vi "Fetch Multi Eval Meas List TPower Results.vi"(8 "error in (no error)":errorcluster, 9 "Result Type (Current)":i32(ring) items=["Current"=0, "Average"=1, "Standard Deviation"=3, "Maximum"=4, "Minimum"=5], 10 "Instance (1)":T1=1, 11 "VISA resource name":refnum<visa-resource-name>) -> (0 "error out":errorcluster, 1 "TPower Results":dbl[](array[numeric]) format="%^.3e", 2 "Reliability":i32, 3 "VISA resource name out":refnum<visa-resource-name>)   [LabVIEW 2015, in "Rohde&Schwarz CMXP NR FR2 Measurement.lvlib"]
doc: "Returns user equipment power values for all measured list mode segments.\n\nAttributes:\nRSCMXPNRFR2M_ATTR_FETCH_MULTI_EVAL_MEASUREMENT_LIST_TPOWER_AVERAGE_RESULTS\nRSCMXPNRFR2M_ATTR_FETCH_MULTI_EVAL_MEASUREMENT_LIST_TPOWER_CURRENT_RESULTS\nRSCMXPNRFR2M_ATTR_FETCH_MULTI_EVAL_MEASUREMENT_LIST_TPOWER_MAXIMUM_RESULTS\nRSCMXPNRFR2M_ATTR_FETCH_MULTI_EVAL_MEASUREMENT_LIST_TPOWER_MINIMUM_RESULTS\nRSCMXPNRFR2M_ATTR_FETCH_MULTI_EVAL_MEASUREMENT_LIST_TPOWER_STANDARD_DEVIATION_RESULTS\n\nRemote-control commands:\nFETCh:NRMMw:MEAS<i>:MEValuation:LIST:MODulation:TPOWer:AVERage?\nFETCh:NRMMw:MEAS<i>:MEValuation:LIST:MODulation:TPOWer:CURRent?\nFETCh:NRMMw:MEAS<i>:MEValuation:LIST:MODulation:TPOWer:MAXimum?\nFETCh:NRMMw:MEAS<i>:MEValuation:LIST:MODulation:TPOWer:MINimum?\nFETCh:NRMMw:MEAS<i>:MEValuation:LIST:MODulation:TPOWer:SDEViation?"
uses:
  <instrlib>/Rohde&Schwarz CMXP NR FR2 Measurement/Rohde&Schwarz CMXP NR FR2 Measurement.lvlib
  <instrlib>/Rohde&Schwarz CMXP NR FR2 Measurement/Private/_Instance.ctl
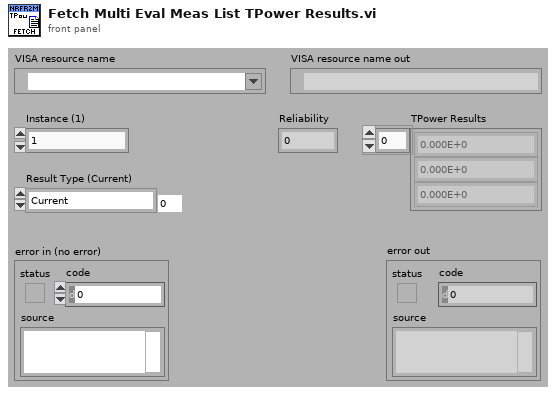
[diagram p1: front panel]
types:
  T1 = typedef "Rohde&Schwarz CMXP NR FR2 Measurement.lvlib/_Instance.ctl" = i32
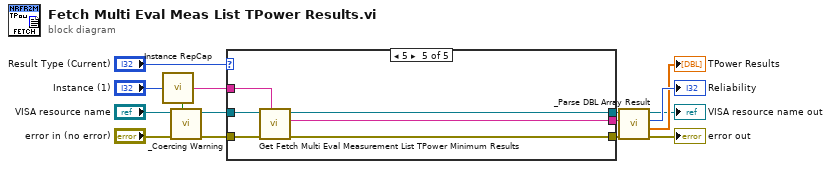
[diagram p0: block diagram]
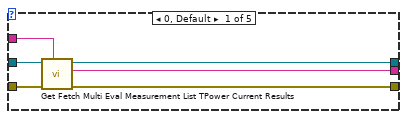
[diagram p2: hidden frame]
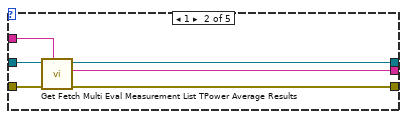
[diagram p3: hidden frame]
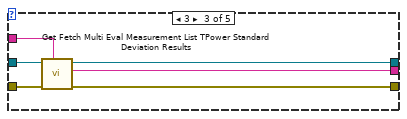
[diagram p4: hidden frame]
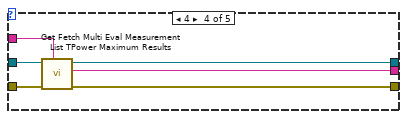
[diagram p5: hidden frame]
diagram:
  n1 = call <instrlib>:"Instance RepCap.vi"("Instance In"="Instance (1)") -> ("In Range?"=w13:bool, "RepCap Identifier Out"=w10:string)  [unwired: 1 in]
  n2 = call <instrlib>:"_Coercing Warning.vi"("In Range?"=w13, "error in (no error)"="error in (no error)", "VISA resource name"="VISA resource name") -> ("error out"=w12:errorcluster, "VISA resource name out"=w11:refnum<visa-resource-name>)  [unwired: 7 in]
  n3 = case shown="5" "Result Type (Current)" {
    tunnel: w12 -> [w21 w27 w33 w39 w45]
    tunnel: w11 -> [w20 w26 w32 w38 w44]
    tunnel: w10 -> [w19 w25 w31 w37 w43]
    tunnel: [w18 w24 w30 w36 w42] -> w8
    tunnel: [w17 w23 w29 w35 w41] -> w7
    tunnel: [w16 w22 w28 w34 w40] -> w6
    frame 0, Default {
      n4 = call "Get Fetch Multi Eval Measurement List TPower Current Results"("Repeated Capabilities"=w19, "error in (no error)"=w21, "instrument handle"=w20) -> ("error out"=w18:errorcluster, "Fetch Multi Eval Measurement List TPower Current Results"=w17:string, "instrument handle out"=w16:refnum<visa-resource-name>)  [unwired: 6 in]
    }
    frame 1 {
      n5 = call "Get Fetch Multi Eval Measurement List TPower Average Results"("Repeated Capabilities"=w25, "error in (no error)"=w27, "instrument handle"=w26) -> ("error out"=w24:errorcluster, "Fetch Multi Eval Measurement List TPower Average Results"=w23:string, "instrument handle out"=w22:refnum<visa-resource-name>)  [unwired: 6 in]
    }
    frame 3 {
      n6 = call "Get Fetch Multi Eval Measurement List TPower Standard Deviation Results"("Repeated Capabilities"=w31, "error in (no error)"=w33, "instrument handle"=w32) -> ("error out"=w30:errorcluster, "Fetch Multi Eval Measurement List TPower Standard Deviation Results"=w29:string, "instrument handle out"=w28:refnum<visa-resource-name>)  [unwired: 6 in]
    }
    frame 4 {
      n7 = call "Get Fetch Multi Eval Measurement List TPower Maximum Results"("Repeated Capabilities"=w37, "error in (no error)"=w39, "instrument handle"=w38) -> ("error out"=w36:errorcluster, "Fetch Multi Eval Measurement List TPower Maximum Results"=w35:string, "instrument handle out"=w34:refnum<visa-resource-name>)  [unwired: 6 in]
    }
    frame 5 {
      n8 = call "Get Fetch Multi Eval Measurement List TPower Minimum Results"("Repeated Capabilities"=w43, "error in (no error)"=w45, "instrument handle"=w44) -> ("error out"=w42:errorcluster, "Fetch Multi Eval Measurement List TPower Minimum Results"=w41:string, "instrument handle out"=w40:refnum<visa-resource-name>)  [unwired: 6 in]
    }
  }
  n9 = call <instrlib>:"_Parse DBL Array Result.vi"("error in (no error)"=w8, "Input String"=w7, "VISA resource name"=w6) -> ("error out"=→"error out":errorcluster, "Results"=→"TPower Results":dbl[], "Reliability"=→"Reliability":i32, "VISA resource name out"=→"VISA resource name out":refnum<visa-resource-name>)  [unwired: 5 in]
